vi "Destroy User Event - Shutdown.vi"(8 "error in (no error)":errorcluster, 11 "User Event - Shutdown":refnum<user-event>) -> (0 "error out":errorcluster)   [LabVIEW 2020, in "User Interface Utilities.lvlib" / "User Event - Shutdown.lvlib"]
doc: "Destroy the user event, even if there is an incoming error."
uses:
  User Event - Shutdown.lvlib
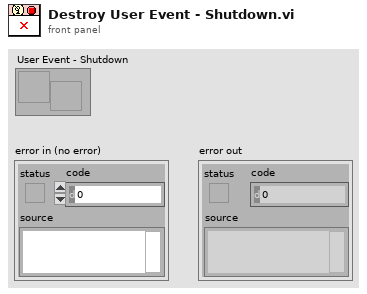
[diagram p1: front panel]
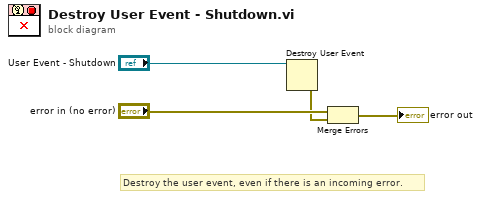
[diagram p0: block diagram]
diagram:
  # "Destroy the user event, even if there is an incoming error."
  n1 = Destroy User Event(user event="User Event - Shutdown") -> (error out=w1:errorcluster)  [unwired: 1 in]
  n2 = Merge Errors("error in (no error)", w1) -> (→"error out":errorcluster)
